vi "MEMR-Process Response.vi"(0 "State In":T1, 5 "Analysis":T2, 7 "Avg":dbl[][](array[numeric]), 9 "Npts":i32) -> (4 "Gain spectra":cluster{"Freq (Hz)":dbl[], "Mag":dbl[][]}[](array[cluster]), 8 "Mag spectra":cluster{"Freq (Hz)":dbl[], dbl[][]}[](array[cluster]))   [LabVIEW 2020]
uses:
  MEMR-Offline Analysis Parameters.ctl
  Typedefs/MEMR-Analysis State.ctl
  Typedefs/MEMR-Analysis.ctl
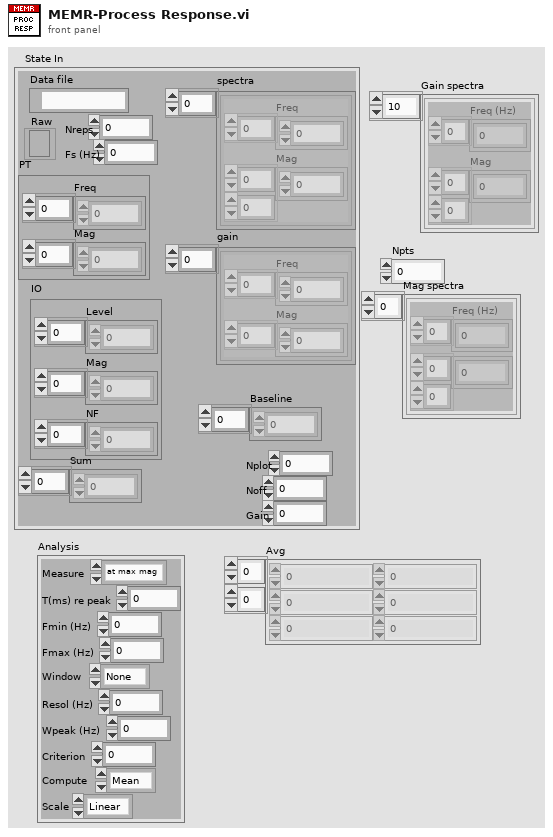
[diagram p1: front panel]
types:
  T1 = typedef "MEMR-Analysis State.ctl" = cluster{"Data file":path, "Raw":refnum<file>, "PT":cluster{"Freq":dbl[], "Mag":dbl[]}, "IO":cluster{"Level":dbl[], "Mag":dbl[], "NF":dbl[]}, "Nreps":i32, "Fs (Hz)":dbl, "Sum":dbl[], "Nplot":i32, "Noff":i32, "Gain":dbl, "spectra":cluster{"Freq":dbl[], "Mag":dbl[][]}[], "gain":cluster{"Freq":dbl[], "Mag":dbl[]}[], "Baseline":dbl[]}
  T2 = typedef "MEMR-Offline Analysis Parameters.ctl" = cluster{"Measure":enum16{"at max mag", "at max gain", "over window", "optimize", "Keefe"}, "T(ms) re peak":dbl, "Fmin (Hz)":dbl, "Fmax (Hz)":dbl, "Window":enum16{"None", "Hanning", "Hamming"}, "Resol (Hz)":dbl, "Wpeak (Hz)":dbl, "Criterion":dbl, "Compute":enum16{"Mean", "Sum"}, "Scale":enum16{"Linear", "Log"}}
  T3 = typedef "MEMR-Analysis.ctl" = cluster{"T(ms) re peak":dbl, "Fmin (Hz)":dbl, "Fmax (Hz)":dbl, "Window":enum16{"None", "Hanning", "Hamming"}, "Gain (dB)":dbl, "Resol (Hz)":dbl}
  T4 = cluster{"Freq (Hz)":dbl[], "+Freq. Mag of FFT (dB rms)":dbl[]}
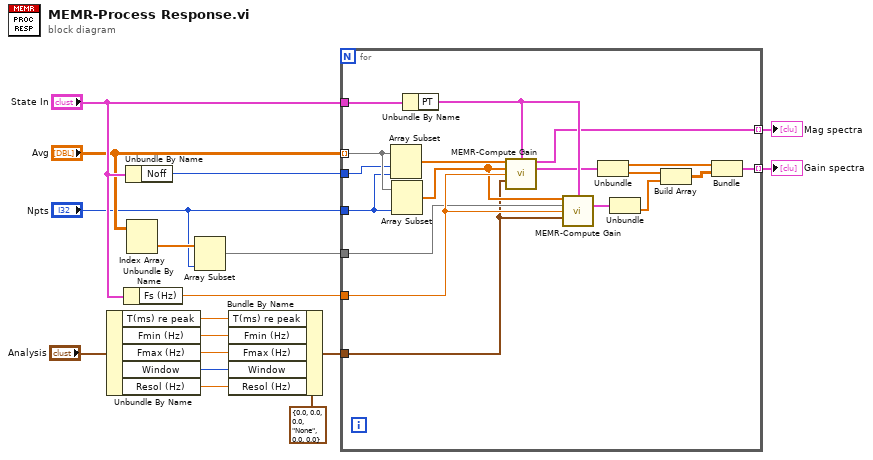
[diagram p0: block diagram]
diagram:
  n1 = Unbundle By Name("Analysis") -> ("T(ms) re peak"=w7:dbl, "Fmin (Hz)"=w6:dbl, "Fmax (Hz)"=w5:dbl, "Window"=w4:enum16{"None", "Hanning", "Hamming"}, "Resol (Hz)"=w3:dbl)
  n2 = Unbundle By Name("State In") -> ("Fs (Hz)"=w15:dbl)
  n3 = Unbundle By Name("State In") -> ("Noff"=w17:i32)
  n4 = Index Array(array="Avg") -> (element=w13:dbl[])  [unwired: 2 in]
  n5 = Array Subset(array=w13, length="Npts") -> (w11:dbl[])  [unwired: 1 in]
  n6 = Bundle By Name(cluster=T3 {"T(ms) re peak"=0.0, "Fmin (Hz)"=0.0, "Fmax (Hz)"=0.0, "Window"=enum."None", "Gain (dB)"=0.0, "Resol (Hz)"=0.0} ("Analysis"), "T(ms) re peak"=w7, "Fmin (Hz)"=w6, "Fmax (Hz)"=w5, "Window"=w4, "Resol (Hz)"=w3) -> (w2:T3)
  n7 = for {
    tunnel: w17 -> [w33]
    tunnel: "Avg" -> [w35] mode=indexing
    tunnel: "Npts" -> [w34]
    tunnel: "State In" -> [w32]
    tunnel: w15 -> [w30]
    tunnel: w11 -> [w28]
    tunnel: [w22] -> w10 mode=indexing
    tunnel: w2 -> [w21]
    tunnel: [w18] -> w1 mode=indexing
    n8 = Array Subset(array=w35, index=w33, length=w34) -> (w31:dbl[])
    n9 = Array Subset(array=w35, length=w34) -> (w29:dbl[])  [unwired: 1 in]
    n10 = Unbundle By Name(w32) -> ("PT"=w27:cluster{"Freq":dbl[], "Mag":dbl[]})
    n11 = call "MEMR-Compute Gain.vi"("Test"=w31, "PT"=w27, "Baseline"=w29, "Fs (Hz)"=w30, "Analysis"=w21) -> ("spectra"=w18:cluster{"Freq (Hz)":dbl[], dbl[][]}, "gain spectrum"=w23:T4)  [unwired: 8 in, 1 out]
    n12 = call "MEMR-Compute Gain.vi"("Test"=w29, "PT"=w27, "Baseline"=w28, "Fs (Hz)"=w30, "Analysis"=w21) -> ("gain spectrum"=w19:T4)  [unwired: 8 in, 2 out]
    n13 = Unbundle(w23) -> ("Freq (Hz)"=w24:dbl[], "+Freq. Mag of FFT (dB rms)"=w20:dbl[])
    n14 = Unbundle(w19) -> ("+Freq. Mag of FFT (dB rms)"=w26:dbl[])  [unwired: 1 out]
    n15 = Build Array(w20, w26) -> (w25:dbl[][])
    n16 = Bundle("Freq (Hz)"=w24, w25) -> (w22:cluster{"Freq (Hz)":dbl[], dbl[][]})  [unwired: 1 in]
  }
  "Gain spectra" <- w10
  "Mag spectra" <- w1
